vi "例4.4.vi"() -> ()   [LabVIEW 2018]
panel:
  in  "y":i8
  in  "x":i8
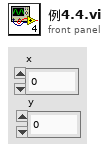
[diagram p1: front panel]
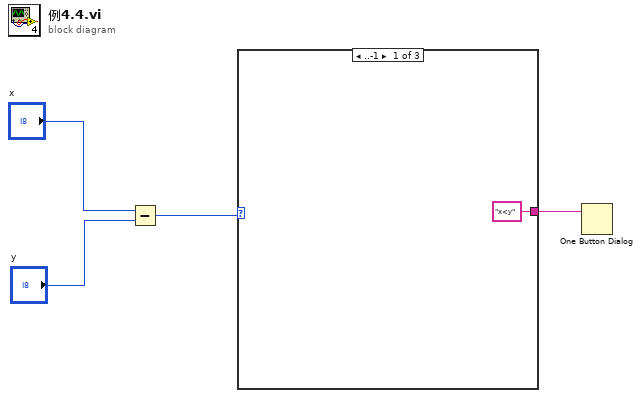
[diagram p0: block diagram]
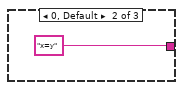
[diagram p2: hidden frame]
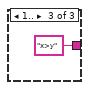
[diagram p3: hidden frame]
diagram:
  n1 = Subtract(x="x", y="y") -> (x-y=w2:i8)
  n2 = case shown="..-1" w2 {
    tunnel: ["x<y" "x=y" "x>y"] -> w1
    frame ..-1 {
    }
    frame 0, Default {
    }
    frame 1.. {
    }
  }
  n3 = One Button Dialog(message=w1) -> ()  [unwired: 1 in, 1 out]
